vi "close handle.vi"(8 "error in (no error)":errorcluster caption="错误输入（无错误）", 11 "http client 输入":refnum<class "http client.lvclass">) -> (0 "error out":errorcluster caption="错误输出", 3 "http client 输出":refnum<class "http client.lvclass">)   [LabVIEW 2016, in "数据传输系统-02.lvlib" / "update.lvlib" / "http client.lvclass"]
uses:
  http client.lvclass
  http client.lvclass/http client.ctl
  <vilib>/httpClient/LabVIEWHTTPClient.lvlib
  update.lvlib
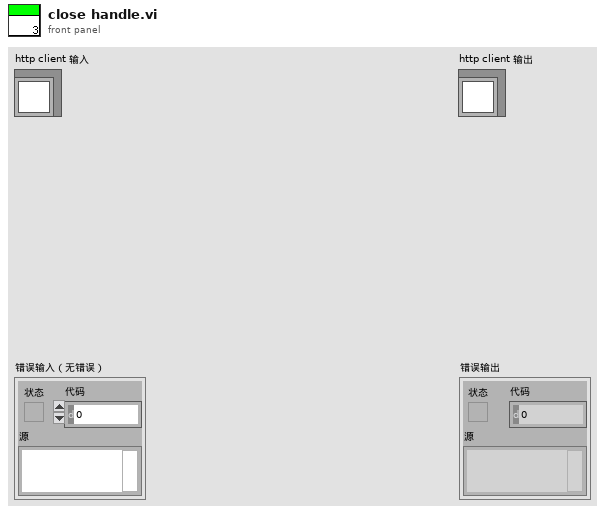
[diagram p1: front panel]
types:
  T1 = typedef "LabVIEWHTTPClient.lvlib/ClientHandle.ctl" = refnum<k1>
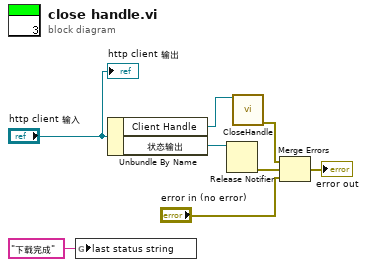
[diagram p0: block diagram]
diagram:
  n1 = global write "更新全局变量.vi" "last status string"("下载完成" ("last status string")) -> ()
  n2 = Unbundle By Name("http client 输入") -> ("Client Handle"=w7:T1, "状态输出"=w6:refnum<notifier>)
  n3 = Release Notifier(notifier=w6) -> (error out=w3:errorcluster)  [unwired: 2 in, 2 out]
  n4 = call <vilib>:"CloseHandle.vi"("client handle"=w7) -> ("error out"=w4:errorcluster)  [unwired: 14 in]
  n5 = Merge Errors(w4, w3, "error in (no error)") -> (→"error out":errorcluster)
  "http client 输出" <- "http client 输入"
